vi "_PC_Daemon_Monitor.vi"(8 "error in (no error)":errorcluster, 11 "Listbox_Ref":refnum<vi>) -> (0 "error out":errorcluster)   [LabVIEW 2018]
uses:
  <vilib>/event_ctls.llb/eventvkey.ctl
  PublicSubVI/Ctl/RegistyFunc.ctl
panel:
  out "XY Graph":cluster{"X":dbl[], "Y":dbl[]}[](graph)
  out "Temperature_turbo":sgl
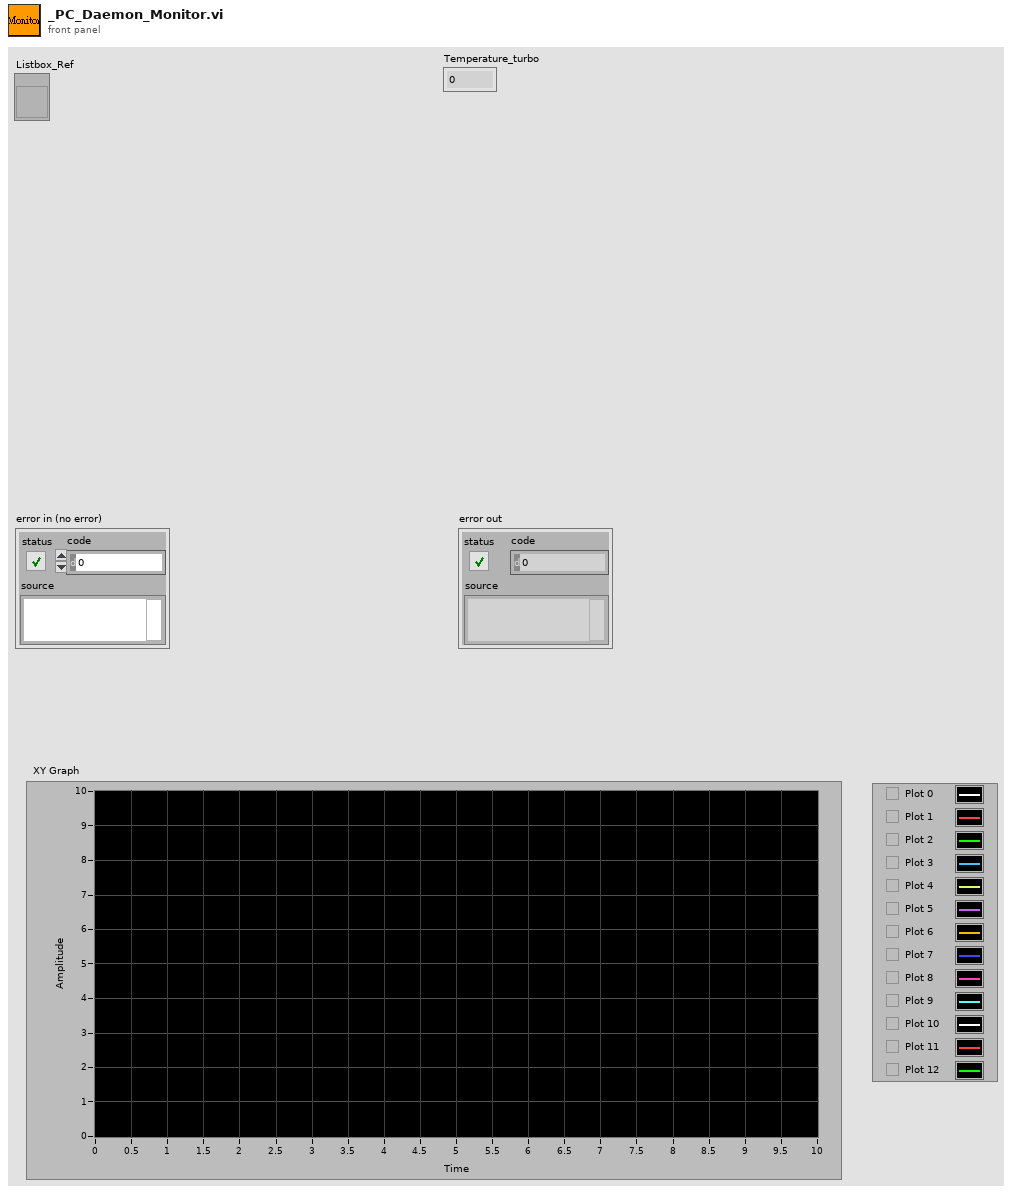
[diagram p1: front panel]
types:
  T1 = typedef "eventvkey.ctl" = enum16{"ASCII", "Enter", "Return", "Shift", "Ctrl", "Alt", "Cmd", "Opt", "Caps", "NumLock", "Clear", "Break", "Up", "Down", "Left", "Right", "Insert", "Delete", "Home", "End", "PageUp", "PageDown", "Escape", "Help", "Pause", "ScrollLock", "F1", "F2", "F3", "F4", "F5", "F6", "F7", "F8", "F9", "F10", "F11", "F12", "F13", "F14", "F15", "F16", "F17", "F18", "F19", "F20", "F21", "F22", "F23", "F24", "Play", "VolumeUp", "VolumeDown", "Mute", "Two Byte Char"}
  T2 = typedef "RegistyFunc.ctl" = enum16{"None", "FileAutoSave", "FileNoise", "FileSN", "ExeStatu", "WorkFolderPath", "MethodPath", "AVGItem", "LoopItem", "AutoRun", "BGColor", "LineColor", "LineWidth", "XGrid", "YGrid", "DeviceRefnum"}
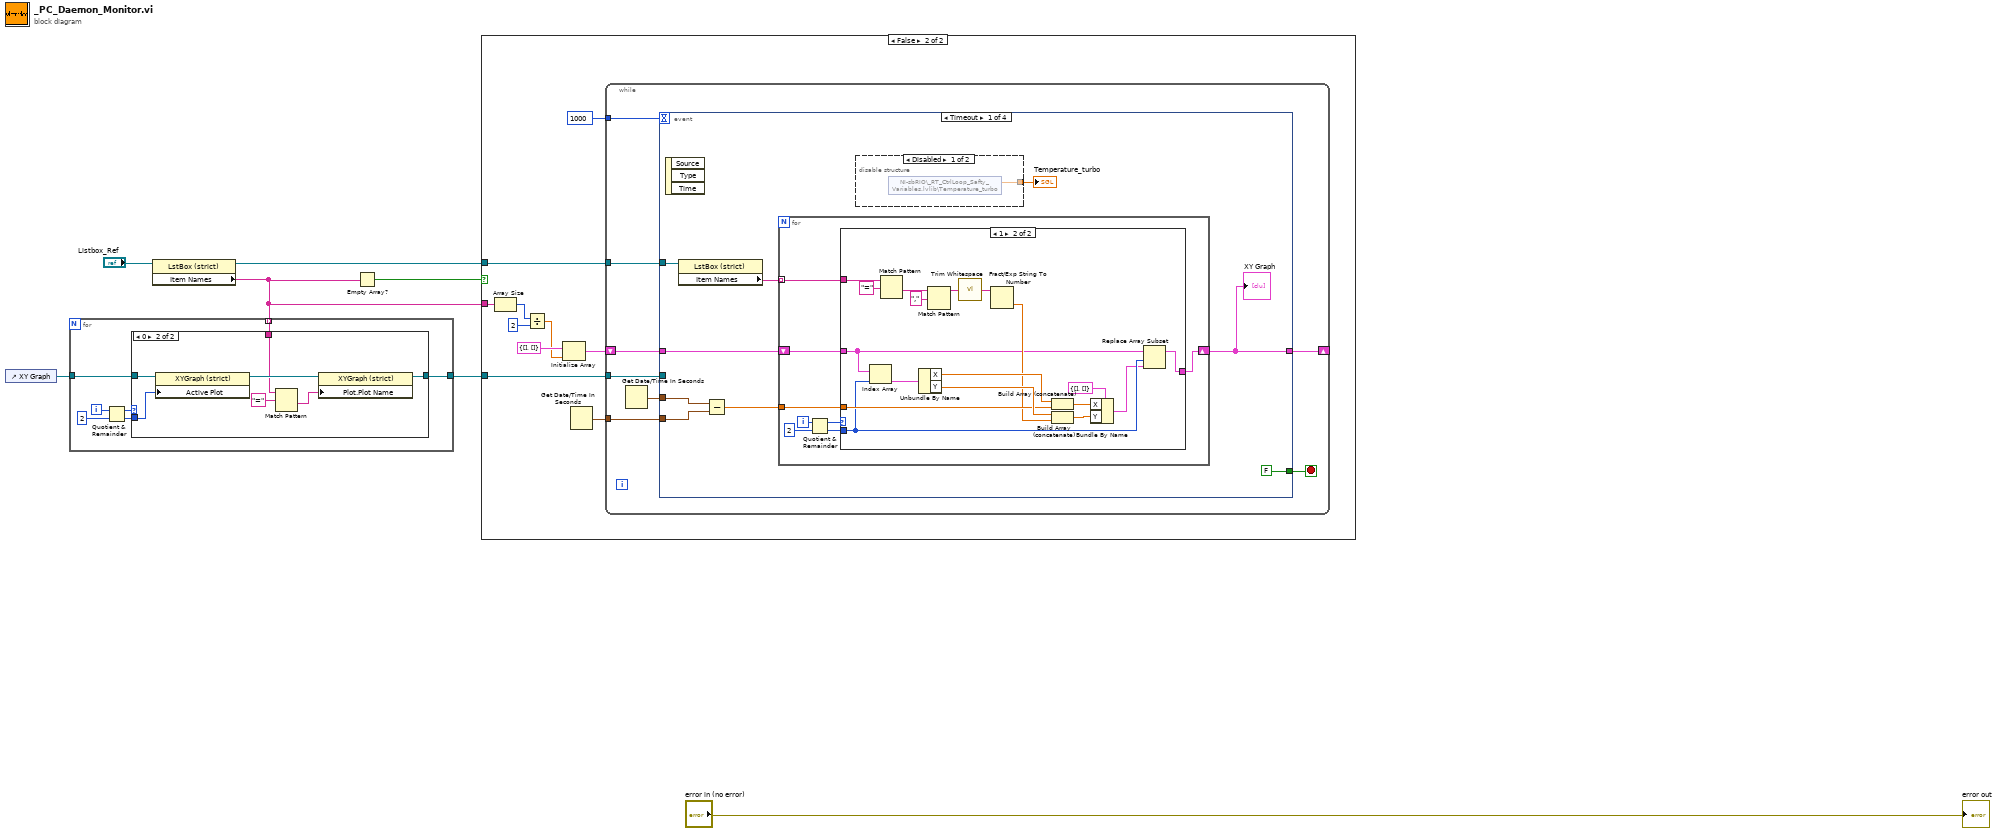
[diagram p0: block diagram]
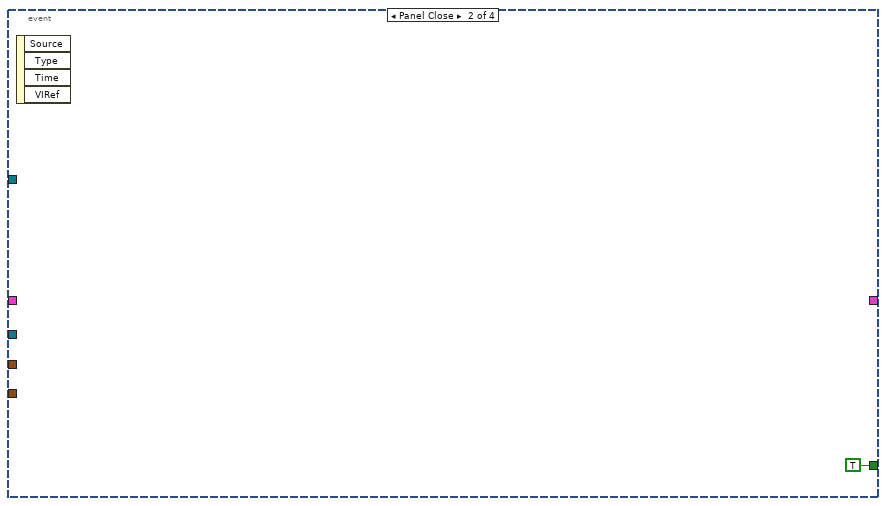
[diagram p5: hidden frame]
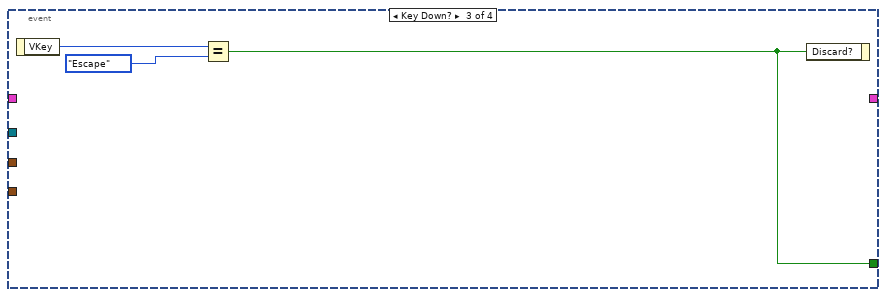
[diagram p6: hidden frame]
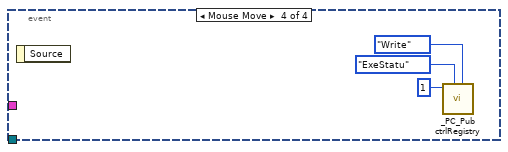
[diagram p7: hidden frame]
diagram:
  n1 = control-ref of="XY Graph"() -> (w4:refnum<vi>)
  n2 = property class="LstBox (strict)"(reference="Listbox_Ref") -> (reference out=w5:refnum<vi>, "Item Names"=w2:string[])  [unwired: 1 in, 1 out]
  n3 = for {
    tunnel: w4 -> [w14]
    tunnel: w2 -> [w9] mode=indexing
    tunnel: [w8] -> w3
    i -> [w12]
    n4 = Quotient & Remainder(x=w12, y=2) -> (x-y*floor(x/y)=w11:i32, floor(x/y)=w10:i32)
    n5 = case shown="0" w11 {
      tunnel: w14 -> [w15 w22]
      tunnel: w10 -> [_ w21]
      tunnel: w9 -> [_ w17]
      tunnel: [w15 w19] -> w8
      frame 1, Default {
      }
      frame 0 {
        n6 = property class="XYGraph (strict)"(reference=w22, "Active Plot"=w21) -> (reference out=w20:refnum<vi>)  [unwired: 1 in, 1 out]
        n7 = Match Pattern(string=w17, regular expression="=") -> (after substring=w16:string)  [unwired: 1 in, 3 out]
        n8 = property class="XYGraph (strict)"(reference=w20, "Plot.Plot Name"=w16) -> (reference out=w19:refnum<vi>)  [unwired: 1 in, 1 out]
      }
    }
  }
  n9 = Empty Array?(array=w2) -> (empty?=w1:bool)
  n10 = case shown="False" w1 {
    tunnel: w5 -> [_ w31]
    tunnel: w3 -> [_ w30]
    tunnel: w2 -> [_ w24]
    frame True {
    }
    frame False {
      n11 = Array Size(array=w24) -> (size(s)=w28:i32)
      n12 = Divide(x=w28, y=2) -> (x/y=w25:dbl)
      n13 = Initialize Array(cluster{"X":dbl[], "Y":dbl[]} {"X"=[], "Y"=[]}, w25) -> (w23:cluster{"X":dbl[], "Y":dbl[]}[])
      n14 = Get Date/Time In Seconds() -> (seconds since 1Jan1904=w29:timestamp)
      n15 = while {
        tunnel: 1000 -> [w40]
        tunnel: w31 -> [w39]
        tunnel: w30 -> [w37]
        tunnel: w29 -> [w36]
        shift-right: [w33] -> _
        shift-left: w23 -> [w34]
        stop <- w38 stop-if-true
        n16 = Get Date/Time In Seconds() -> (seconds since 1Jan1904=w35:timestamp)
        n17 = event shown="[0] Timeout" {
          selector: _ -> [_ _ _ _]
          dyn-events: _ -> [_ _ _ _]
          timeout: w40 -> [_ _ _ _]
          tunnel: w39 -> [w48 _ _ _]
          tunnel: [FALSE TRUE w79 _] -> w38
          tunnel: w37 -> [_ _ _ _]
          tunnel: w36 -> [w45 _ _ _]
          tunnel: w35 -> [w46 _ _ _]
          tunnel: w34 -> [w42 _ _ _]
          tunnel: [w41 _ _ _] -> w33
          event Timeout {
            n18 = event-data() -> ()  [unwired: 1 in, 3 out]
            n19 = property class="LstBox (strict)"(reference=w48) -> ("Item Names"=w47:string[])  [unwired: 1 in, 2 out]
            n20 = Subtract(x=w46, y=w45) -> (x-y=w44:dbl)
            n21 = for {
              tunnel: w47 -> [w54] mode=indexing
              tunnel: w44 -> [w52]
              shift-right: [w51] -> w41
              shift-left: w42 -> [w53]
              i -> [w58]
              n22 = Quotient & Remainder(x=w58, y=2) -> (x-y*floor(x/y)=w56:i32, floor(x/y)=w55:i32)
              n23 = case shown="1" w56 {
                tunnel: w55 -> [_ w62]
                tunnel: w54 -> [_ w74]
                tunnel: w53 -> [w59 w63]
                tunnel: w52 -> [_ w67]
                tunnel: [w59 w60] -> w51
                frame 0, Default {
                }
                frame 1 {
                  n24 = Index Array(array=w63, index=w62) -> (element=w70:cluster{"X":dbl[], "Y":dbl[]})
                  n25 = Match Pattern(string=w74, regular expression="=") -> (after substring=w73:string)  [unwired: 1 in, 3 out]
                  n26 = Unbundle By Name(w70) -> ("X"=w69:dbl[], "Y"=w68:dbl[])
                  n27 = Match Pattern(string=w73, regular expression=",") -> (before substring=w76:string)  [unwired: 1 in, 3 out]
                  n28 = call <vilib>:"Trim Whitespace.vi"("string"=w76) -> ("trimmed string"=w72:string)  [unwired: 1 in]
                  n29 = Fract/Exp String To Number(string=w72) -> (number=w66:dbl)  [unwired: 3 in, 1 out]
                  n30 = Build Array (concatenate)(w69, w67) -> (w65:dbl[])
                  n31 = Build Array (concatenate)(w68, w66) -> (w64:dbl[])
                  n32 = Bundle By Name(cluster=cluster{"X":dbl[], "Y":dbl[]} {"X"=[], "Y"=[]} ("element"), "X"=w65, "Y"=w64) -> (w61:cluster{"X":dbl[], "Y":dbl[]})
                  n33 = Replace Array Subset(array=w63, new element=w61, index=w62) -> (w60:cluster{"X":dbl[], "Y":dbl[]}[])
                }
              }
            }
            "XY Graph" <- w41
            n34 = disable-structure shown="Disabled" {
              disable-tunnel: [w50 _] -> w49
              frame Disabled {
                n35 = shared-variable "NI-sbRIO\\_RT_CtrlLoop_Safty_Variables.lvlib\\Temperature_turbo"() -> (w50:sgl)  [unwired: 1 in, 1 out]
              }
              frame Enabled {
              }
            }
            "Temperature_turbo" <- w49
          }
          event Panel Close {
            n36 = event-data() -> ()  [unwired: 1 in, 4 out]
          }
          event Key Down? {
            n37 = event-data() -> ("VKey"=w81:T1)  [unwired: 1 in]
            n38 = Equal?(x=w81, y=eventvkey."Escape") -> (x = y?=w79:bool)
            n39 = event-data("Discard?"=w79) -> ()  [unwired: 1 in, 1 out]
          }
          event Mouse Move {
            n40 = event-data() -> ()  [unwired: 1 in, 1 out]
            n41 = call "_PC_Pub ctrlRegistry.vi"("type"=enum16{"None", "Write", "Read"}."Write", "function"=RegistyFunc."ExeStatu", "write value"=u32 1) -> ()  [unwired: 5 in, 4 out]
          }
        }
      }
    }
  }
  "error out" <- "error in (no error)"
